vi "nevstop-programming-palette - Pre-Build Custom Action.vi"(10 "Variant":variant) -> (0 "error out":errorcluster)   [LabVIEW 2017]
panel:
  out "n":i32
  out "i":i32
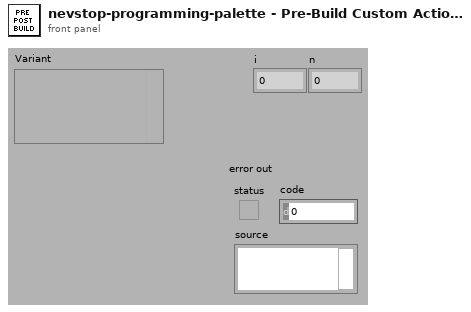
[diagram p1: front panel]
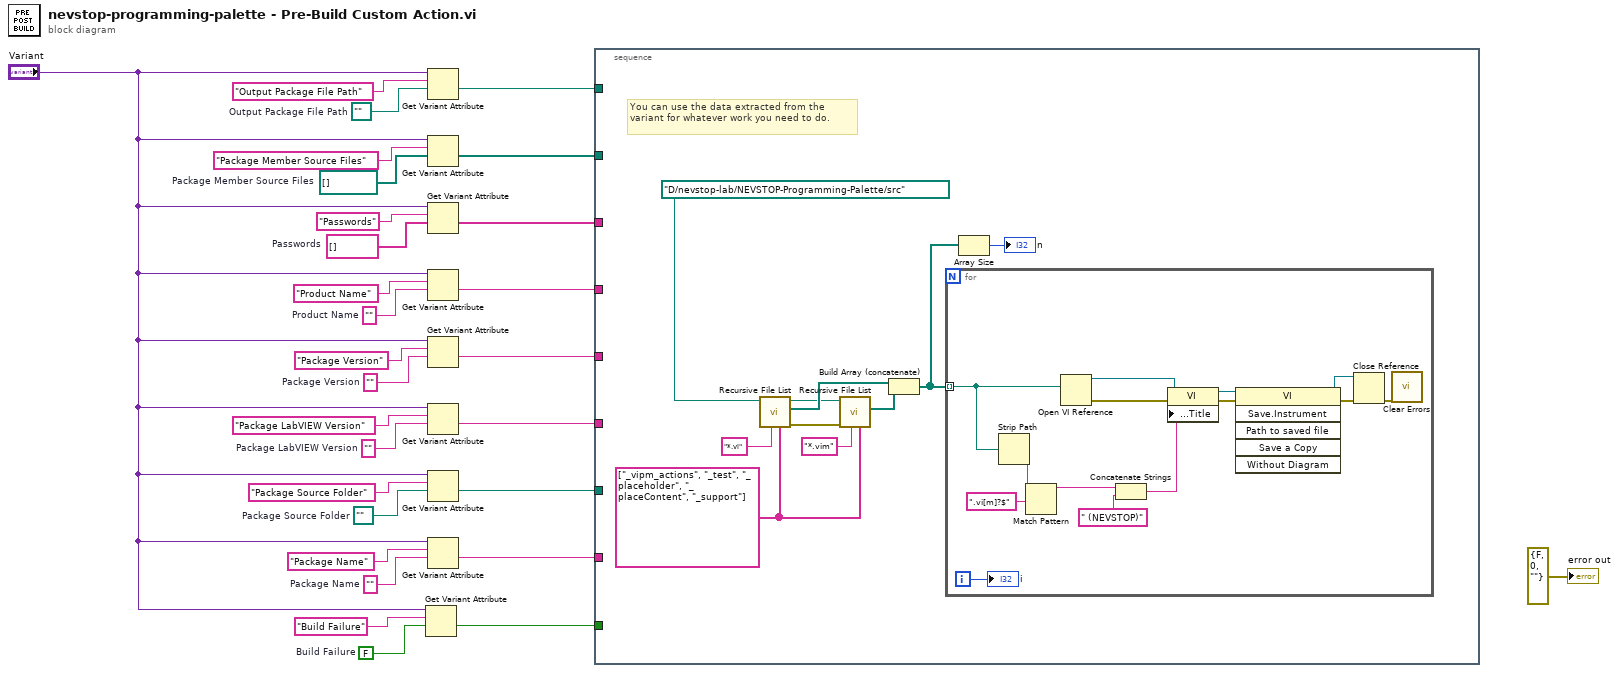
[diagram p0: block diagram]
diagram:
  w3 = FALSE  # Build Failure
  w13 = path ""  # Package Source Folder
  w14 = ""  # Package Name
  w17 = ""  # Package LabVIEW Version
  w19 = ""  # Package Version
  w21 = ""  # Product Name
  w24 = string[] []  # Passwords
  w26 = path[] []  # Package Member Source Files
  w28 = path ""  # Output Package File Path
  n1 = Get Variant Attribute(Variant="Variant", name="Build Failure", default value (empty Variant)=w3) -> (value=w1:bool)  [unwired: 1 in, 3 out]
  n2 = Get Variant Attribute(Variant="Variant", name="Output Package File Path", default value (empty Variant)=w28) -> (value=w12:path)  [unwired: 1 in, 3 out]
  n3 = Get Variant Attribute(Variant="Variant", name="Package Member Source Files", default value (empty Variant)=w26) -> (value=w11:path[])  [unwired: 1 in, 3 out]
  n4 = Get Variant Attribute(Variant="Variant", name="Passwords", default value (empty Variant)=w24) -> (value=w10:string[])  [unwired: 1 in, 3 out]
  n5 = Get Variant Attribute(Variant="Variant", name="Product Name", default value (empty Variant)=w21) -> (value=w9:string)  [unwired: 1 in, 3 out]
  n6 = Get Variant Attribute(Variant="Variant", name="Package Version", default value (empty Variant)=w19) -> (value=w8:string)  [unwired: 1 in, 3 out]
  n7 = Get Variant Attribute(Variant="Variant", name="Package LabVIEW Version", default value (empty Variant)=w17) -> (value=w7:string)  [unwired: 1 in, 3 out]
  n8 = Get Variant Attribute(Variant="Variant", name="Package Source Folder", default value (empty Variant)=w13) -> (value=w6:path)  [unwired: 1 in, 3 out]
  n9 = Get Variant Attribute(Variant="Variant", name="Package Name", default value (empty Variant)=w14) -> (value=w5:string)  [unwired: 1 in, 3 out]
  n10 = stacked-sequence {
    tunnel: w12 -> [_]
    tunnel: w11 -> [_]
    tunnel: w10 -> [_]
    tunnel: w9 -> [_]
    tunnel: w8 -> [_]
    tunnel: w7 -> [_]
    tunnel: w6 -> [_]
    tunnel: w5 -> [_]
    tunnel: w1 -> [_]
    frame #0 {
      w32 = string[] ["_vipm_actions", "_test", "_placeholder", "_placeContent", "_support"] ("Folders to Exclude")
      # "You can use the data extracted from the variant for whatever work you need to do."
      n11 = call <vilib>:"Recursive File List.vi"("Folders to Exclude"=w32, "pattern"="*.vi", "Folder Path"=path "D:/nevstop-lab/NEVSTOP-Programming-Palette/src") -> ("error out"=w37:errorcluster, "All Files in Dir"=w36:path[], "dup Folder Path"=w33:path)  [unwired: 4 in, 2 out]
      n12 = call <vilib>:"Recursive File List.vi"("Folders to Exclude"=w32, "pattern"="*.vim", "error in (no error)"=w37, "Folder Path"=w33) -> ("All Files in Dir"=w35:path[])  [unwired: 3 in, 4 out]
      n13 = Build Array (concatenate)(w36, w35) -> (w31:path[])
      n14 = for {
        tunnel: w31 -> [w47] mode=indexing
        i -> [w41]
        n15 = Strip Path(path=w47) -> (name=w46:string)  [unwired: 1 out]
        n16 = Match Pattern(string=w46, regular expression=".vi[m]?$") -> (before substring=w44:string)  [unwired: 1 in, 3 out]
        n17 = Open VI Reference(vi path=w47) -> (vi reference=w53:refnum<vi>, error out=w48:errorcluster)  [unwired: 5 in]
        n18 = Concatenate Strings(w44, " (NEVSTOP)" ("string")) -> (w43:string)
        n19 = property class="VI"(reference=w53, error in=w48, "Front Panel.Title"=w43) -> (reference out=w52:refnum<vi>, error out=w51:errorcluster)
        n20 = invoke class="VI" method="Save.Instrument"(reference=w52, error in=w51) -> (reference out=w49:refnum<vi>, error out=w50:errorcluster)  [unwired: 4 in, 4 out]
        n21 = Close Reference(reference=w49, error in (no error)=w50) -> (error out=w40:errorcluster)
        n22 = call <vilib>:"Clear Errors.vi"("error in (no error)"=w40) -> ()  [unwired: 5 in, 2 out]
        "i" <- w41
      }
      n23 = Array Size(array=w31) -> (size(s)=→"n":i32)
    }
  }
  "error out" <- errorcluster {"status"=FALSE, "code"=0, "source"=""} ("error out")
